vi "FGV_PROXY_DIAGNOSTICS_records_display.vi"(4 "front_panel_reference":refnum<vi>, 6 "SQL_listbox_reference":refnum<vi>, 7 "options":T3, 8 "error_in":errorcluster, 9 "station":T1, 11 "input":variant) -> (0 "error_out":errorcluster, 1 "all_info":T2)   [LabVIEW 2020]
uses:
  FGV_PROXY_DIAGNOSTICS_records_display.ctl
  PROXY_DIAGNOSTICS_all_info.ctl
  STATION/station.ctl
  ini/typedef/PROXY_all_config_info.ctl
  ini/typedef/PROXY_main_ini_file.ctl
  queues/typedef/PROXY_queue_refnums.ctl
  queues/typedef/STATION_queue_element.ctl
  STATION/ST_SQL_sequence_state.ctl
  _misc/PLC_connection_status.ctl
  DIAGNOSTICS_connection_indicators/FGV_PROXY_connection_indicators.ctl
  _misc/AULocalize/SubVIs/Get Localized Phrase Compact Interface 1D.vi
  _misc/AULocalize/SubVIs/Get Localized Phrase Compact Interface 0D.vi
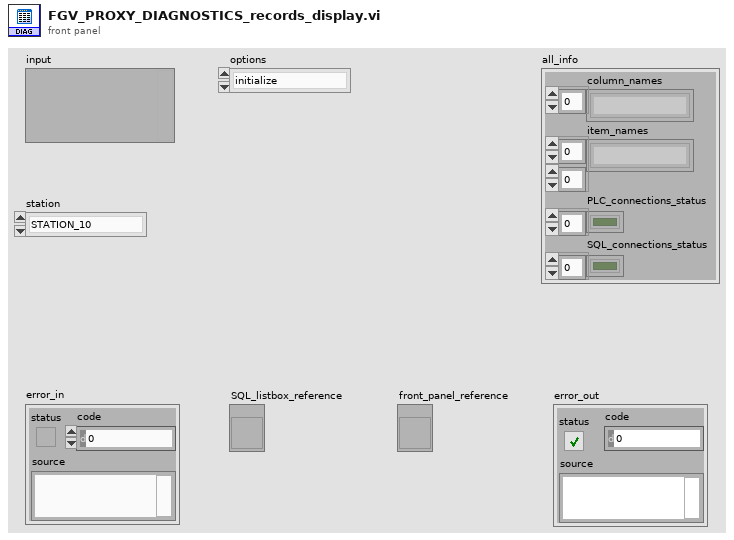
[diagram p1: front panel]
types:
  T1 = typedef "station.ctl" = enum16{"STATION_10", "STATION_20", "STATION_30", "STATION_40", "STATION_50", "STATION_60", "STATION_70", "STATION_80", "STATION_90", "STATION_100", "STATION_110", "STATION_120", "STATION_165", "MAIN"}
  T2 = typedef "PROXY_DIAGNOSTICS_all_info.ctl" = cluster{"column_names":string[], "item_names":string[][], "PLC_connections_status":bool[], "SQL_connections_status":bool[]}
  T3 = typedef "FGV_PROXY_DIAGNOSTICS_records_display.ctl" = enum16{"initialize", "set_PLC_IP", "set_PLC_Port", "set_PLC_connection_status", "set_SQL_connection_status", "get_all_info"}
  T4 = typedef "PROXY_all_config_info.ctl" = cluster{"main_ini_file":T5, "SQL Password":string, "queue_refnums":T6, "number_of_stations":i32}
  T5 = typedef "PROXY_main_ini_file.ctl" = cluster{"SQL Driver":string, "SQL Server":string, "SQL Database":string, "SQL UID":string, "Reference table":string, "Reference history":string, "Archivisation CFG table":string, "Archivisation CFG history":string, "User table":string, "User history":string, "default language":string, "REF CHG listener IP":string, "REF CHG listener port":u16, "ST 10 name":string, "ST 10 listener IP":string, "ST 10 listener port":u16, "ST 20 name":string, "ST 20 listener IP":string, "ST 20 listener port":u16, "ST 30 name":string, "ST 30 listener IP":string, "ST 30 listener port":u16, "ST 40 name":string, "ST 40 listener IP":string, "ST 40 listener port":u16, "ST 50 name":string, "ST 50 listener IP":string, "ST 50 listener port":u16, "ST 60 name":string, "ST 60 listener IP":string, "ST 60 listener port":u16, "ST 70 name":string, "ST 70 listener IP":string, "ST 70 listener port":u16, "ST 80 name":string, "ST 80 listener IP":string, "ST 80 listener port":u16, "ST 90 name":string, "ST 90 listener IP":string, "ST 90 listener port":u16, "ST 100 name":string, "ST 100 listener IP":string, "ST 100 listener port":u16, "ST 110 name":string, "ST 110 listener IP":string, "ST 110 listener port":u16, "ST 120 name":string, "ST 120 listener IP":string, "ST 120 listener port":u16, "ST 165 name":string, "ST 165 listener IP":string, "ST 165 listener port":u16}
  T6 = typedef "PROXY_queue_refnums.ctl" = cluster{"ST_10_queue":refnum<queue>, "ST_20_queue":refnum<queue>, "ST_30_queue":refnum<queue>, "ST_40_queue":refnum<queue>, "ST_50_queue":refnum<queue>, "ST_60_queue":refnum<queue>, "ST_70_queue":refnum<queue>, "ST_80_queue":refnum<queue>, "ST_90_queue":refnum<queue>, "ST_100_queue":refnum<queue>, "ST_110_queue":refnum<queue>, "ST_120_queue":refnum<queue>, "ST_165_queue":refnum<queue>}
  T7 = typedef "FGV_PROXY_connection_indicators.ctl" = enum16{"initialize", "SQL_conn_ind_update", "PLC_conn_ind_update"}
  T8 = typedef "PLC_connection_status.ctl" = enum16{"Connected", "Waiting", "Error", "-"}
  T9 = cluster{"station":T1, "disabled index (col)":i32}
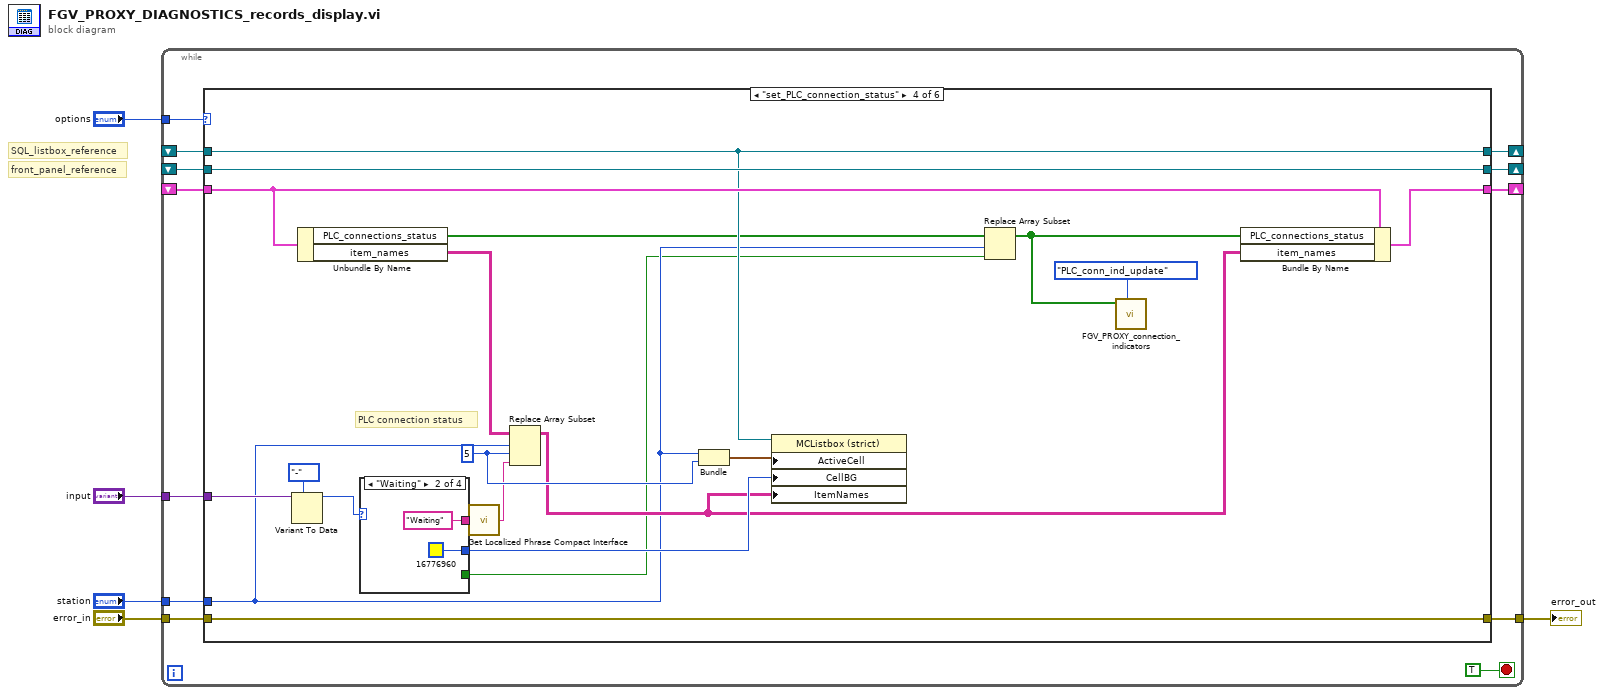
[diagram p0: block diagram]
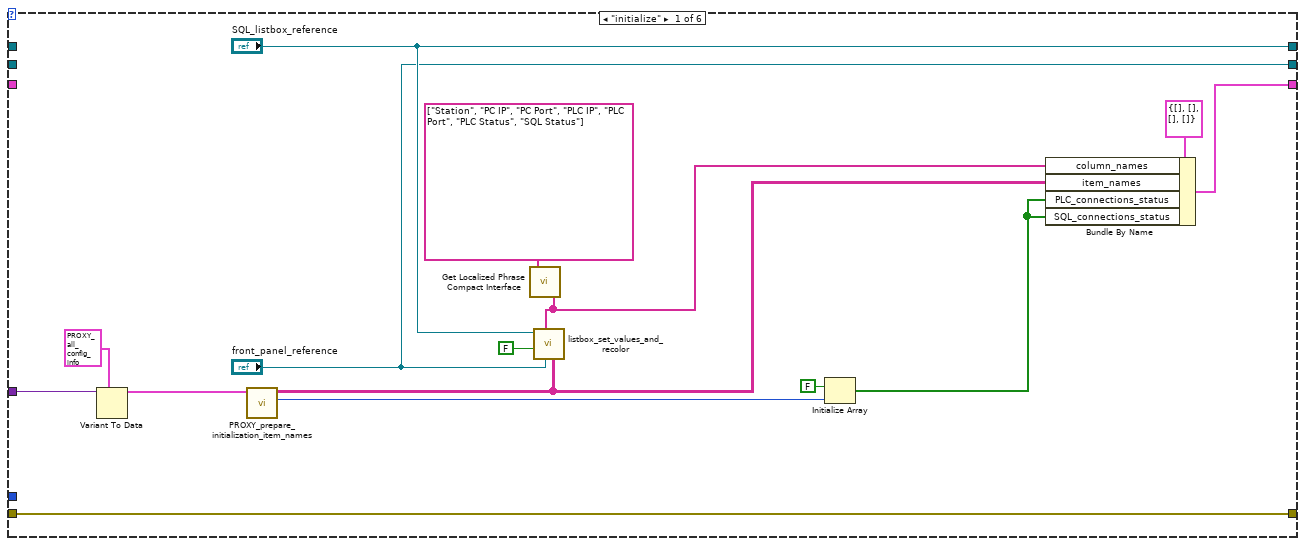
[diagram p2: hidden frame]
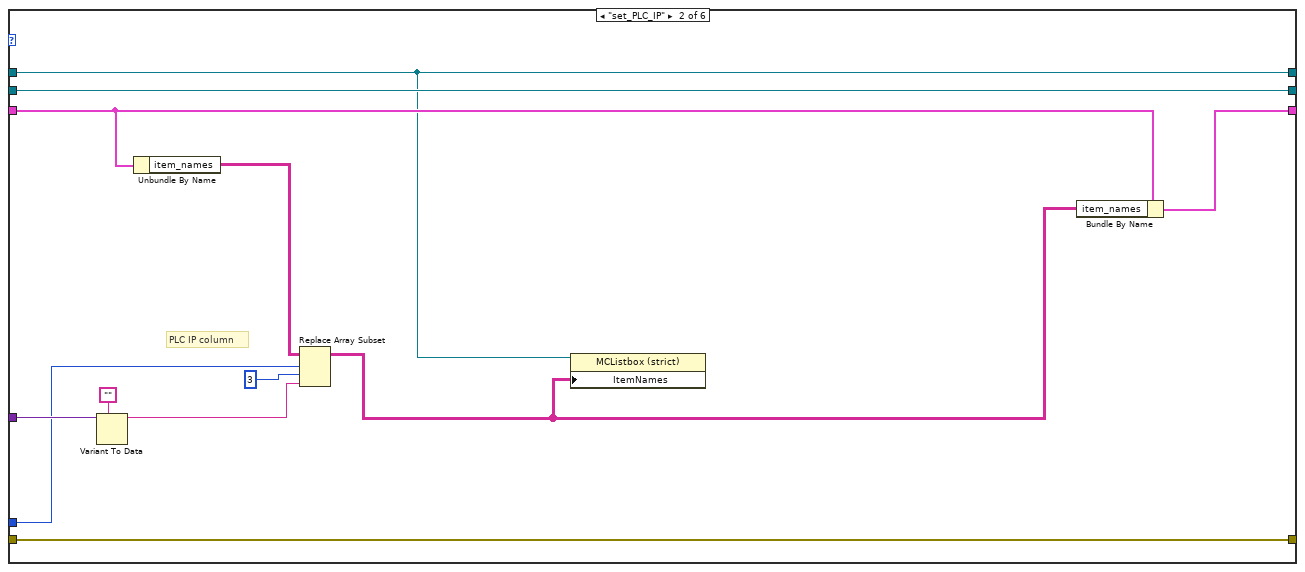
[diagram p3: hidden frame]
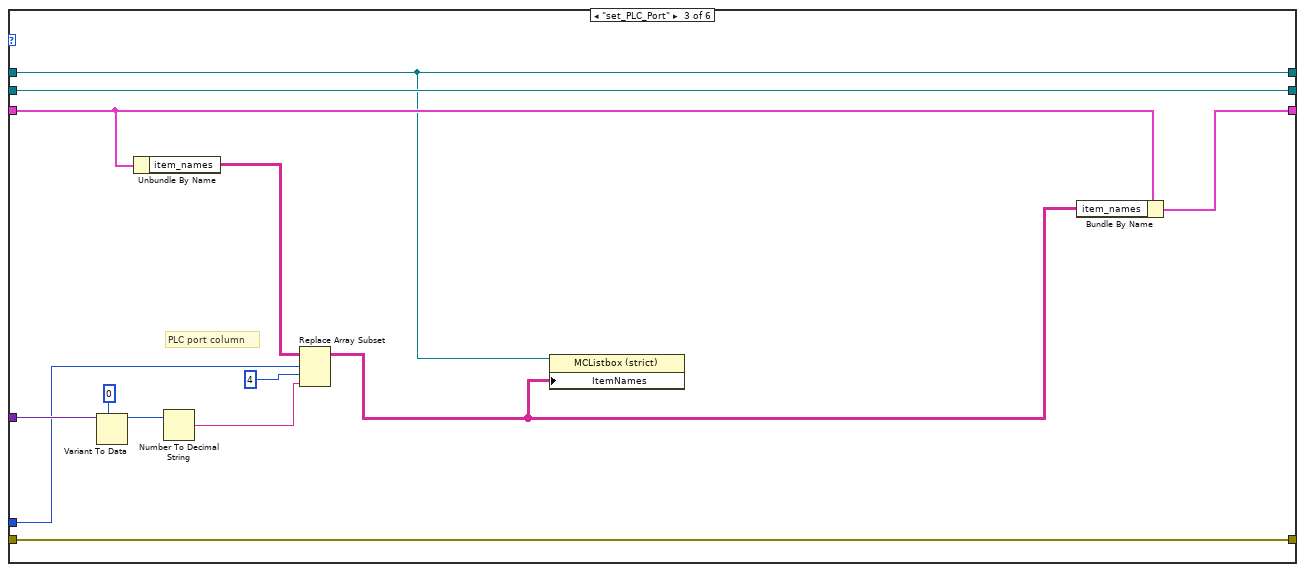
[diagram p4: hidden frame]
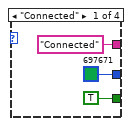
[diagram p5: hidden frame]
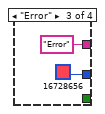
[diagram p6: hidden frame]
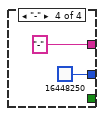
[diagram p7: hidden frame]
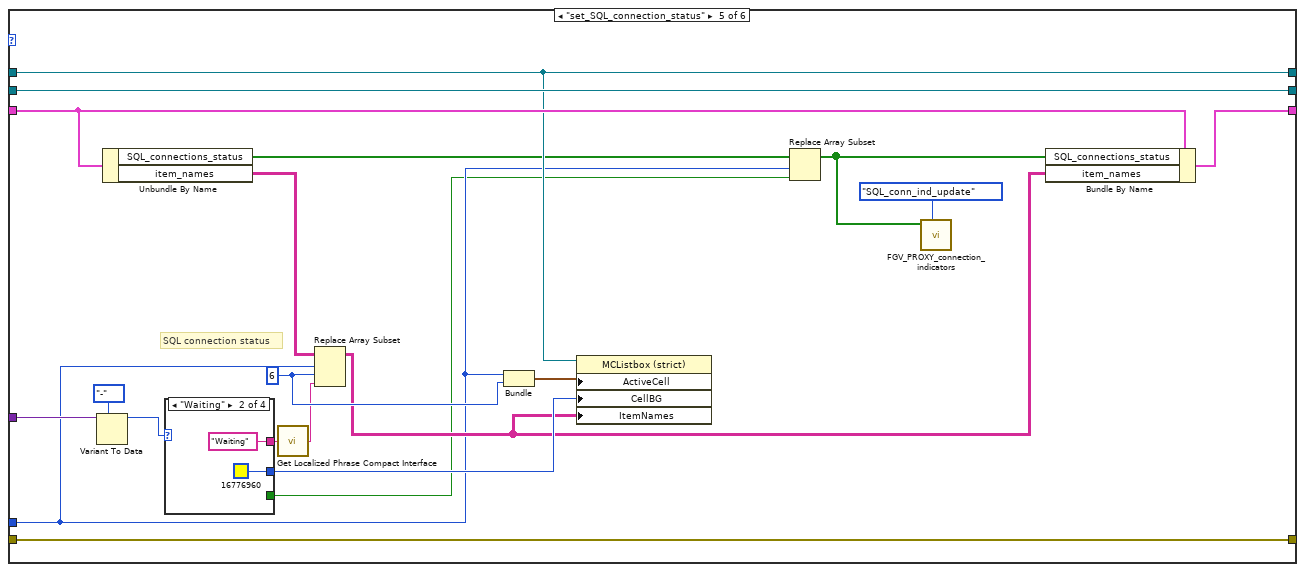
[diagram p8: hidden frame]
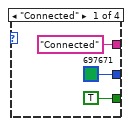
[diagram p9: hidden frame]
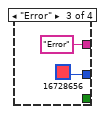
[diagram p10: hidden frame]
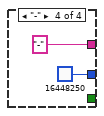
[diagram p11: hidden frame]
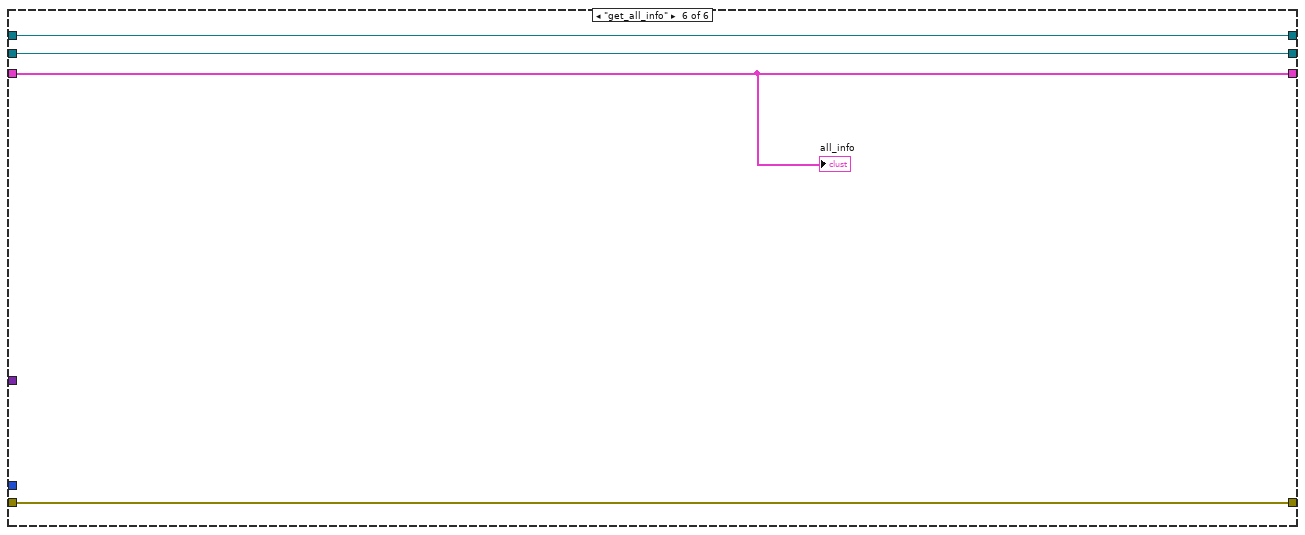
[diagram p12: hidden frame]
diagram:
  # "front_panel_reference"
  # "SQL_listbox_reference"
  n1 = while {
    tunnel: "options" -> [w16]
    tunnel: [w15] -> w5
    tunnel: "error_in" -> [w14]
    shift-right: [w13] -> _
    shift-left: _ -> [w12]
    shift-right: [w11] -> _
    shift-left: _ -> [w10]
    tunnel: "input" -> [w9]
    shift-right: [w8] -> _
    shift-left: _ -> [w7]
    tunnel: "station" -> [w6]
    stop <- TRUE stop-if-true
    n2 = case shown="\"set_PLC_connection_status\"" w16 {
      tunnel: [w32 w44 w57 w77 w106 w118] -> w15
      tunnel: w14 -> [w32 w44 w57 w77 w106 w118]
      tunnel: [w25 w42 w55 w75 w104 w119] -> w13
      tunnel: w12 -> [_ w41 w54 w74 w103 w119]
      tunnel: ["SQL_listbox_reference" w34 w46 w65 w94 w117] -> w11
      tunnel: w10 -> [_ w34 w46 w65 w94 w117]
      tunnel: w9 -> [w29 w43 w56 w76 w105 _]
      tunnel: ["front_panel_reference" w35 w47 w66 w95 w116] -> w8
      tunnel: w7 -> [_ w35 w47 w66 w95 w116]
      tunnel: w6 -> [_ w37 w52 w62 w91 _]
      frame "initialize" {
        n3 = Variant To Data(type=T4 {"main_ini_file"={"SQL Driver"="", "SQL Server"="", "SQL Database"="", "SQL UID"="", "Reference table"="", "Reference history"="", "Archivisation CFG table"="", "Archivisation CFG history"="", "User table"="", "User history"="", "default language"="", "REF CHG listener IP"="", "REF CHG listener port"=0, "ST 10 name"="", "ST 10 listener IP"="", "ST 10 listener port"=0, "ST 20 name"="", "ST 20 listener IP"="", "ST 20 listener port"=0, "ST 30 name"="", "ST 30 listener IP"="", "ST 30 listener port"=0, "ST 40 name"="", "ST 40 listener IP"="", "ST 40 listener port"=0, "ST 50 name"="", "ST 50 listener IP"="", "ST 50 listener port"=0, "ST 60 name"="", "ST 60 listener IP"="", "ST 60 listener port"=0, "ST 70 name"="", "ST 70 listener IP"="", "ST 70 listener port"=0, "ST 80 name"="", "ST 80 listener IP"="", "ST 80 listener port"=0, "ST 90 name"="", "ST 90 listener IP"="", "ST 90 listener port"=0, "ST 100 name"="", "ST 100 listener IP"="", "ST 100 listener port"=0, "ST 110 name"="", "ST 110 listener IP"="", "ST 110 listener port"=0, "ST 120 name"="", "ST 120 listener IP"="", "ST 120 listener port"=0, "ST 165 name"="", "ST 165 listener IP"="", "ST 165 listener port"=0}, "SQL Password"="", "queue_refnums"={"ST_10_queue"=refnum, "ST_20_queue"=refnum, "ST_30_queue"=refnum, "ST_40_queue"=refnum, "ST_50_queue"=refnum, "ST_60_queue"=refnum, "ST_70_queue"=refnum, "ST_80_queue"=refnum, "ST_90_queue"=refnum, "ST_100_queue"=refnum, "ST_110_queue"=refnum, "ST_120_queue"=refnum, "ST_165_queue"=refnum}, "number_of_stations"=0} ("all_config_info"), Variant=w29) -> (data=w27:T4)  [unwired: 1 in, 1 out]
        n4 = call "PROXY_prepare_initialization_item_names.vi"("all_config_info"=w27) -> ("number_of_stations"=w21:i32, "item_names"=w23:string[][])  [unwired: 9 in]
        n5 = call-poly "Get Localized Phrase Compact Interface.vi"("Key"=string[] ["Station", "PC IP", "PC Port", "PLC IP", "PLC Port", "PLC Status", "SQL Status"] ("column_names")) -> ("Translated Phrase"=w18:string[])
        n6 = call "listbox_set_values_and_recolor.vi"("item_names"=w23, "front_panel_reference"="front_panel_reference", "column_names"=w18, "Autosize? (T)"=FALSE, "multicolumn_listbox_reference_in"="SQL_listbox_reference") -> ()  [unwired: 5 in, 2 out]
        n7 = Initialize Array(FALSE, w21) -> (w19:bool[])
        n8 = Bundle By Name(cluster=T2 {"column_names"=[], "item_names"=[], "PLC_connections_status"=[], "SQL_connections_status"=[]} ("SQL_selection"), "column_names"=w18, "item_names"=w23, "PLC_connections_status"=w19, "SQL_connections_status"=w19) -> (w25:T2)
      }
      frame "set_PLC_IP" {
        # "PLC IP column"
        n9 = Variant To Data(type="", Variant=w43) -> (data=w38:string)  [unwired: 1 in, 1 out]
        n10 = Unbundle By Name(w41) -> ("item_names"=w39:string[][])
        n11 = Replace Array Subset(array=w39, new element=w38, index (row)=w37, index (col)=3 ("disabled index (col)")) -> (w33:string[][])
        n12 = property class="MCListbox (strict)"(reference=w34, "ItemNames"=w33) -> ()  [unwired: 1 in, 2 out]
        n13 = Bundle By Name(cluster=w41, "item_names"=w33) -> (w42:T2)
      }
      frame "set_PLC_Port" {
        # "PLC port column"
        n14 = Variant To Data(type=u16 0 ("remote port"), Variant=w56) -> (data=w49:u16)  [unwired: 1 in, 1 out]
        n15 = Unbundle By Name(w54) -> ("item_names"=w53:string[][])
        n16 = Number To Decimal String(number=w49) -> (decimal integer string=w48:string)  [unwired: 1 in]
        n17 = Replace Array Subset(array=w53, new element=w48, index (row)=w52, index (col)=4 ("disabled index (col)")) -> (w45:string[][])
        n18 = property class="MCListbox (strict)"(reference=w46, "ItemNames"=w45) -> ()  [unwired: 1 in, 2 out]
        n19 = Bundle By Name(cluster=w54, "item_names"=w45) -> (w55:T2)
      }
      frame "set_PLC_connection_status" {
        w67 = 5 ("disabled index (col)")
        # "PLC connection status"
        n20 = Variant To Data(type=PLC_connection_status."-", Variant=w76) -> (data=w71:T8)  [unwired: 1 in, 1 out]
        n21 = Unbundle By Name(w74) -> ("PLC_connections_status"=w63:bool[], "item_names"=w73:string[][])
        n22 = case shown="\"Waiting\"" w71 {
          tunnel: ["Connected" "Waiting" "Error" "-"] -> w70
          tunnel: [u32 697671 u32 16776960 u32 16728656 u32 16448250] -> w69
          tunnel: [TRUE _ _ _] -> w61
          frame "Connected" {
          }
          frame "Waiting" {
          }
          frame "Error" {
          }
          frame "-" {
          }
        }
        n23 = call-poly "Get Localized Phrase Compact Interface.vi"("Key"=w70) -> ("Translated Phrase"=w58:string)
        n24 = Replace Array Subset(array=w73, new element=w58, index (row)=w62, index (col)=w67) -> (w64:string[][])
        n25 = Bundle("station"=w62, "disabled index (col)"=w67) -> (w68:T9)  [unwired: 1 in]
        n26 = property class="MCListbox (strict)"(reference=w65, "ActiveCell"=w68, "CellBG"=w69, "ItemNames"=w64) -> ()  [unwired: 1 in, 2 out]
        n27 = Replace Array Subset(array=w63, new element=w61, index=w62) -> (w59:bool[])
        n28 = call "FGV_PROXY_connection_indicators.vi"("options"=FGV_PROXY_connection_indicators."PLC_conn_ind_update", "status_array"=w59) -> ()  [unwired: 9 in, 1 out]
        n29 = Bundle By Name(cluster=w74, "PLC_connections_status"=w59, "item_names"=w64) -> (w75:T2)
      }
      frame "set_SQL_connection_status" {
        w96 = 6 ("disabled index (col)")
        # "SQL connection status"
        n30 = Variant To Data(type=PLC_connection_status."-", Variant=w105) -> (data=w100:T8)  [unwired: 1 in, 1 out]
        n31 = Unbundle By Name(w103) -> ("SQL_connections_status"=w92:bool[], "item_names"=w102:string[][])
        n32 = case shown="\"Waiting\"" w100 {
          tunnel: ["Connected" "Waiting" "Error" "-"] -> w99
          tunnel: [u32 697671 u32 16776960 u32 16728656 u32 16448250] -> w98
          tunnel: [TRUE _ _ _] -> w90
          frame "Connected" {
          }
          frame "Waiting" {
          }
          frame "Error" {
          }
          frame "-" {
          }
        }
        n33 = call-poly "Get Localized Phrase Compact Interface.vi"("Key"=w99) -> ("Translated Phrase"=w87:string)
        n34 = Replace Array Subset(array=w102, new element=w87, index (row)=w91, index (col)=w96) -> (w93:string[][])
        n35 = Bundle("station"=w91, "disabled index (col)"=w96) -> (w97:T9)  [unwired: 1 in]
        n36 = property class="MCListbox (strict)"(reference=w94, "ActiveCell"=w97, "CellBG"=w98, "ItemNames"=w93) -> ()  [unwired: 1 in, 2 out]
        n37 = Replace Array Subset(array=w92, new element=w90, index=w91) -> (w88:bool[])
        n38 = call "FGV_PROXY_connection_indicators.vi"("options"=FGV_PROXY_connection_indicators."SQL_conn_ind_update", "status_array"=w88) -> ()  [unwired: 9 in, 1 out]
        n39 = Bundle By Name(cluster=w103, "SQL_connections_status"=w88, "item_names"=w93) -> (w104:T2)
      }
      frame "get_all_info" {
        "all_info" <- w119
      }
    }
  }
  "error_out" <- w5
